vi "Line Detector.vi"(6 "milliseconds to wait":u32=100, 8 "error in":errorcluster, 9 "kena brp":dbl, 10 "Speed":dbl=250.0, 11 "FPGA VI Reference Out 2":refnum<k20>) -> (0 "error out":errorcluster, 2 "STOP?":bool, 3 "FPGA VI Reference Out":refnum<k20>)   [LabVIEW 2019]
uses:
  <vilib>/Platform/TimedLoop/XDataNode/timing_clust.ctl
  <vilib>/Platform/TimedLoop/XDataNode/nitl_modes.ctl
  <vilib>/Platform/TimedLoop/XDataNode/wakeup.ctl
  <vilib>/robotics/Steering/Mecanum Wheel/Roller Orientation.ctl
  <vilib>/robotics/Steering/Wheel/Wheel Parameters.ctl
  <vilib>/robotics/Steering/Wheel/Rotation Direction.ctl
  <vilib>/robotics/Steering/Mecanum Steering Frame/NI_Robotics_Mecanum Steering Frame.lvclass
  C:/Program Files (x86)/National Instruments/LabVIEW 2019/vi.lib/robotics/Steering/Steering Frame/NI_Robotics_Steering Frame.lvclass
  <vilib>/robotics/Steering/Mecanum Wheel/Create Mecanum Wheel.vi
  <vilib>/robotics/Steering/Mecanum Steering Frame/Create Mecanum Steering Frame.vi
  <vilib>/Utility/error.llb/Error Cluster From Error Code.vi
  <vilib>/rvi/errors/niLvFpgaAdjustHostInterfaceError.vi
  <vilib>/robotics/Steering/Steering Frame/Apply Steering Frame Velocity to Motors.vi
  <vilib>/platform/TimedLoop/XDataNode/XDataNode.xnode
  <vilib>/robotics/Steering/Create Steering Frame/NI_Robotics_Create Steering Frame.xnode
  <vilib>/robotics/Steering/Class Type Definitions/Mecanum Steering Frame.ctl
  <vilib>/rvi/interface/nirviReadWriteControl/nirviReadWriteControl.xnode
  <vilib>/robotics/Steering/Steering Frame/NI_Robotics_Steering Frame.lvclass
  NiFpgaLv.dll
  <vilib>/rvi/interface/Simulation/niFpgaSimulationCallBeginRW.vi
  <vilib>/Platform/TimedLoop/XDataNode/XDNodeRunTimeDep.lvlib
  <vilib>/robotics/Steering/Class Type Definitions/NI_Robotics_Steering Class Types.lvlib
  <vilib>/robotics/Steering/Wheel/NI_Robotics_Wheel.lvclass
  <vilib>/robotics/Steering/Mecanum Wheel/NI_Robotics_Mecanum Wheel.lvclass
  C:/Program Files (x86)/National Instruments/LabVIEW 2019/vi.lib/robotics/Steering/Special Steering Frame/NI_Robotics_Special Steering Frame.lvclass
  <vilib>/rvi/interface/nirviOpenFPGA/nirviOpenFPGA.xnode
  Collin's Project/FPGA Bitfiles/MRmecanum_FPGATarget_FPGAMainModified_TerasRobot_LKSN2021.lvbitx
  <vilib>/FPGAPlugInAG/myRIO-1900/niLvFpga_Open_myRIO-1900.vi
  <vilib>/rvi/interface/common/dynamic/niFpgaDynamicAddResources.vi
panel:
  out "Reset Button":bool
  out "LINE 2":bool
  out "LINE 1":bool
  out "now":dbl
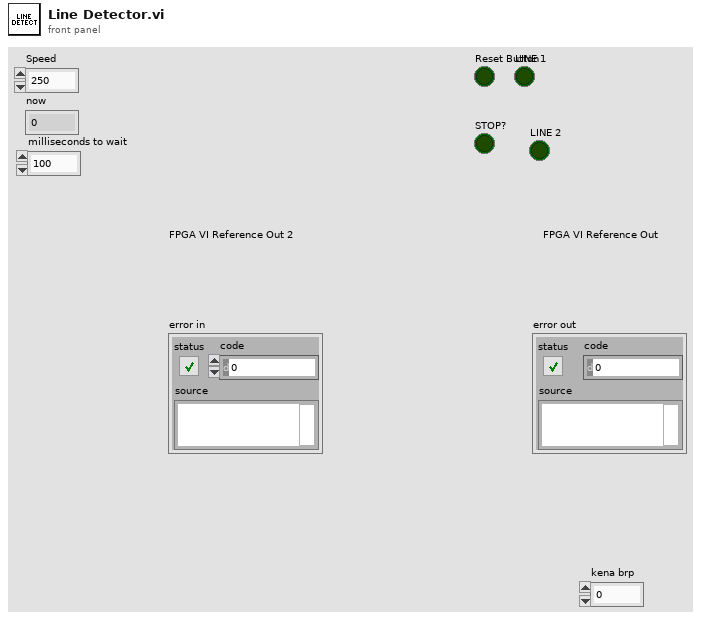
[diagram p1: front panel]
types:
  T1 = enum16{"maju", "mundur", "kanan", "kiri", "atas kanan", "atas kiri", "bawah kanan", "bawah kiri", "putar kanan", "putar kiri"}
  T2 = typedef "NI_Robotics_Steering Class Types.lvlib/Mecanum Steering Frame.ctl" = refnum<class "NI_Robotics_Mecanum Steering Frame.lvclass">
  T3 = typedef "XDNodeRunTimeDep.lvlib/timing_clust.ctl" = cluster{"Expected End [f-1]":u64, "Actual End [f-1]":u64, "Finished Late? [f-1]":bool, "Expected End [i-1]":u64, "Actual End [i-1]":u64, "Finished Late? [i-1]":bool, "Expected Start [i]":u64, "Actual Start [i]":u64, "Expected Start [f]":u64, "Actual Start [f]":u64, "Source Name":string, "Structure Name":string, "Period":i64, "Deadline":i64, "Offset":i64, "Start":i64, "Priority":i32, "Timeout":i32, "Mode":T4, "Wakeup Reason":T5, "Error":errorcluster, "Source Type":string, "Secondary Source Type":string, "Global End Time":u64, "Global Start Time":u64, "Frame Duration":u64, "Iteration Duration":u64, "Assigned CPU":i32, "I/O Scan Engine Mode":u32}
  T4 = typedef "XDNodeRunTimeDep.lvlib/nitl_modes.ctl" = enum32{"No Change", "Process missed periods, maintain original phase", "Discard missed periods, maintain original phase", "Process missed periods, ignore original phase", "Discard missed periods, ignore original phase"}
  T5 = typedef "XDNodeRunTimeDep.lvlib/wakeup.ctl" = enum32{"Normal", "Aborted", "Asynchronous wakeup", "Timing source error", "Timed loop error", "Timeout"}
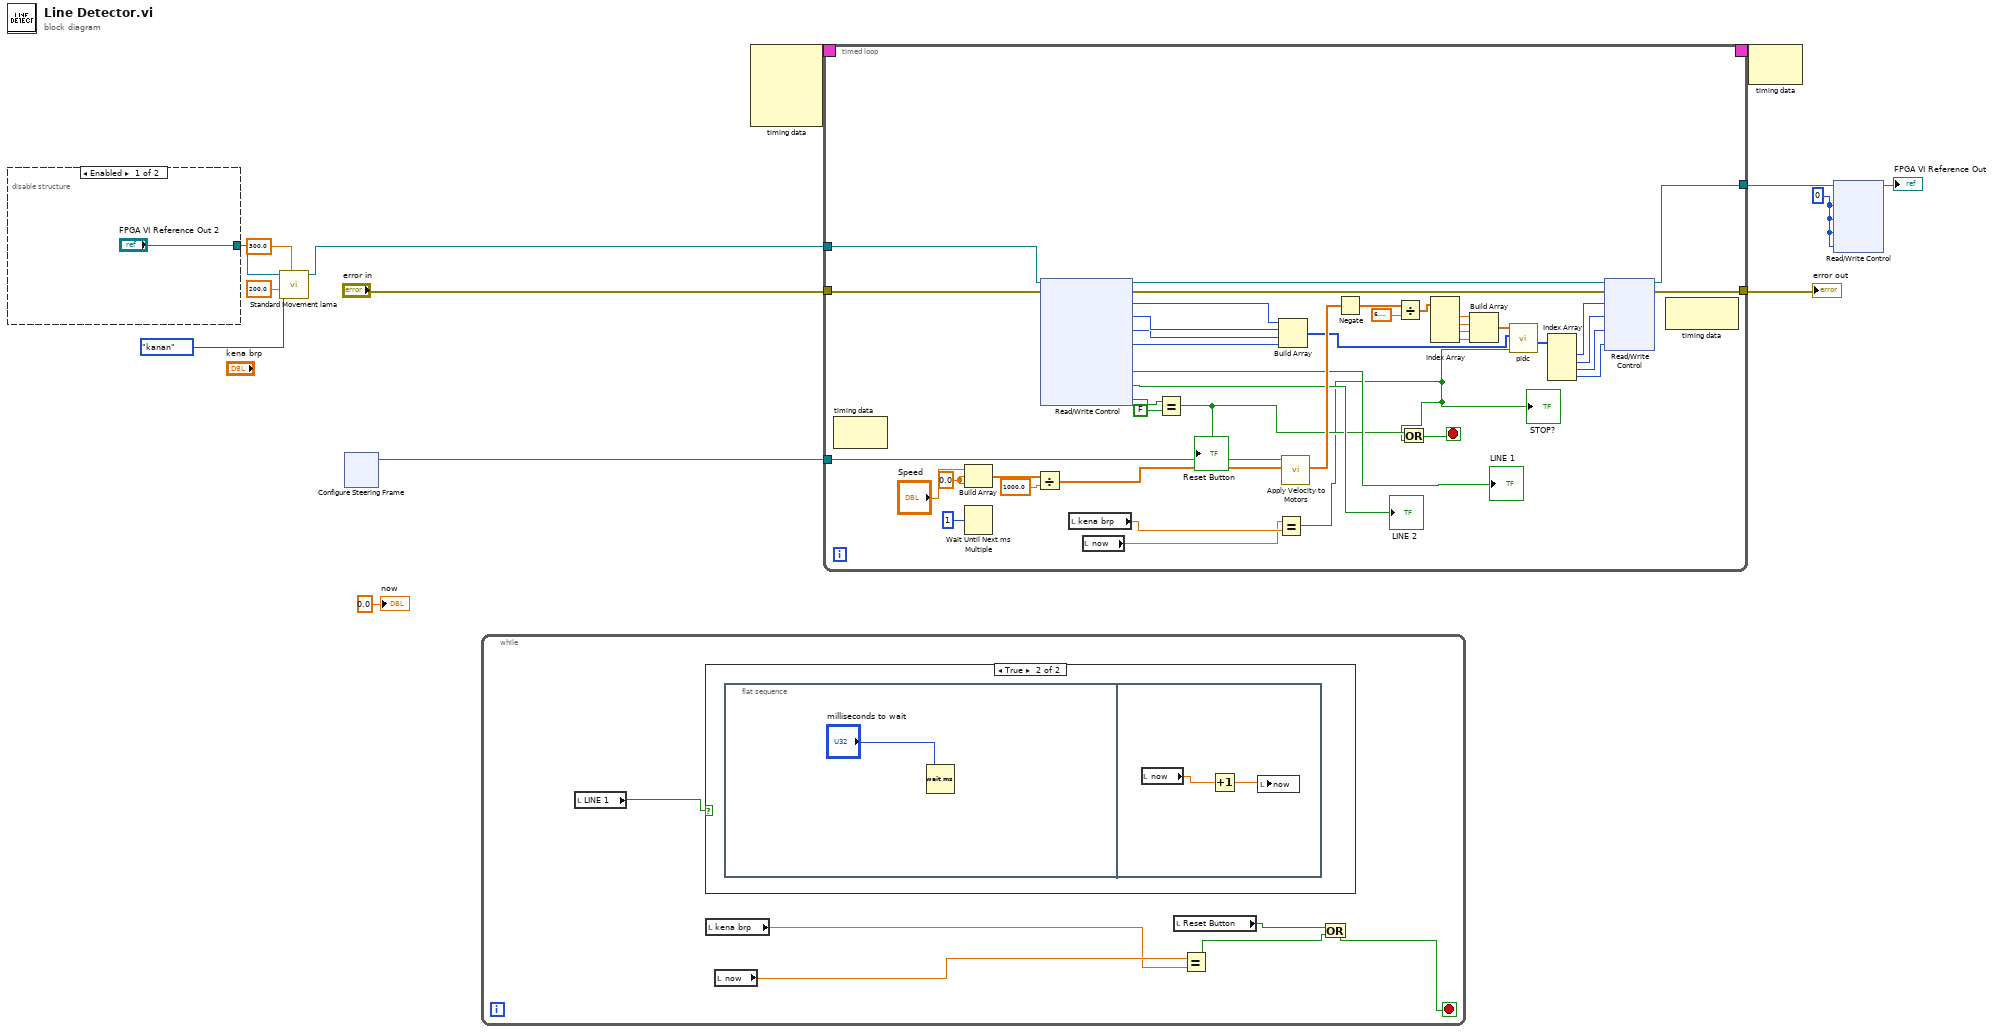
[diagram p0: block diagram]
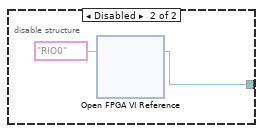
[diagram p3: hidden frame]
diagram:
  w7 = i16 0 ("M3")
  n1 = disable-structure shown="Enabled" {
    disable-tunnel: ["FPGA VI Reference Out 2" w16] -> w5
    frame Enabled {
    }
    frame Disabled {
      n2 = xnode "Open FPGA VI Reference"("resource name"=tag "RIO0") -> ("FPGA VI Reference Out"=w16:refnum<k20>)  [unwired: 1 in, 1 out]
    }
  }
  n3 = call "Standard Movement lama.vi"("Time"=300.0, "Speed"=200.0, "Move"=T1."kanan", "FPGA VI Reference Out 2"=w5) -> ("FPGA VI Reference Out"=w4:refnum<k20>)  [unwired: 6 in, 1 out]
  n4 = xnode ("Configure Steering Frame")() -> ("mecanum steering frame out"=w11:T2)  [unwired: 1 in, 1 out]
  n5 = while {
    stop <- w18 stop-if-true
    n6 = local read "LINE 1"() -> (w21:bool)
    n7 = case shown="True" w21 {
      frame False {
      }
      frame True {
        n8 = flat-sequence {
          frame #0 {
            n9 = Wait (ms)(milliseconds to wait="milliseconds to wait") -> ()  [unwired: 1 out]
          }
          frame #1 {
            n10 = local read "now"() -> (w26:dbl)
            n11 = Increment(x=w26) -> (x+1=w25:dbl)
            n12 = local write "now"(w25) -> ()
          }
        }
      }
    }
    n13 = local read "kena brp"() -> (w22:dbl)
    n14 = local read "now"() -> (w23:dbl)
    n15 = local read "Reset Button"() -> (w20:bool)
    n16 = Equal?(x=w23, y=w22) -> (x = y?=w19:bool)
    n17 = Or(x=w20, y=w19) -> (x .or. y?=w18:bool)
  }
  n18 = node-c288() -> (w13:T3)  [unwired: 4 in]
  n19 = timed-loop {
    timing: w13 -> [_]
    timing-out: [_] -> w12
    tunnel: w11 -> [w67]
    tunnel: w4 -> [w64]
    tunnel: [w66] -> w9
    tunnel: "error in" -> [w63]
    tunnel: [w65] -> w14
    stop <- w27 stop-if-true
    w37 = 0.0 ("element")
    n20 = node-c288() -> ()  [unwired: 1 in, 1 out]
    n21 = Build Array("Speed", w37, w37) -> (w41:dbl[])
    n22 = Wait Until Next ms Multiple(millisecond multiple=u32 1) -> ()  [unwired: 1 out]
    n23 = Divide(x=w41, y=1000.0) -> (x/y=w42:dbl[])
    n24 = xnode "Read/Write Control"("FPGA VI Reference In"=w64, "error in"=w63) -> ("FPGA VI Reference Out"=w36:refnum<k20>, "error out"=w61:errorcluster, "ENC M1"=w53:i32, "ENC M2"=w52:i32, "ENC M3"=w51:i32, "ENC M4"=w50:i32, "LINE 1"=→"LINE 1":bool, "LINE 2"=→"LINE 2":bool, "START BUTTON"=w31:bool)  [unwired: 1 out]
    n25 = local read "kena brp"() -> (w35:dbl)
    n26 = local read "now"() -> (w34:dbl)
    n27 = Equal?(x=w31, y=FALSE) -> (x = y?=w29:bool)
    "Reset Button" <- w29
    n28 = Equal?(x=w34, y=w35) -> (x = y?=w28:bool)
    "STOP?" <- w28
    n29 = Build Array(w53, w52, w51, w50) -> (w49:i32[])
    n30 = call-poly <vilib>:"Apply Velocity to Motors.vi"("steering frame velocity"=w42, "steering frame in"=w67) -> ("ccw motor velocity setpoints"=w62:dbl[])  [unwired: 5 in, 4 out]
    n31 = Negate(x=w62) -> (-x=w60:dbl[])
    n32 = Divide(x=w60, y=6.283185307179586) -> (x/y=w58:dbl[])
    n33 = Or(x=w29, y=w28) -> (x .or. y?=w27:bool)
    n34 = Index Array(array=w58) -> (element #1=w57:dbl, element #2=w56:dbl, element #3=w55:dbl, element #4=w54:dbl)  [unwired: 4 in]
    n35 = Build Array(w57, w56, w55, w54) -> (w48:dbl[])
    n36 = call "pidc.vi"("Stop"=w28, "input encoder 2"=w49, "input rps"=w48) -> ("Output duty cycle"=w47:i16[])  [unwired: 8 in]
    n37 = Index Array(array=w47) -> (element #1=w46:i16, element #2=w45:i16, element #3=w44:i16, element #4=w43:i16)  [unwired: 4 in]
    n38 = xnode "Read/Write Control"("FPGA VI Reference In"=w36, "error in"=w61, "M1"=w46, "M2"=w45, "M3"=w44, "M4"=w43) -> ("FPGA VI Reference Out"=w66:refnum<k20>, "error out"=w65:errorcluster)
    n39 = node-c288() -> ()  [unwired: 1 in, 1 out]
  }
  "error out" <- w14
  n40 = node-c288(w12) -> ()  [unwired: 1 out]
  n41 = xnode "Read/Write Control"("FPGA VI Reference In"=w9, "M3"=w7, "M1"=w7, "M4"=w7, "M2"=w7) -> ("FPGA VI Reference Out"=→"FPGA VI Reference Out":refnum<k20>)  [unwired: 1 in, 1 out]
  "now" <- 0.0 ("now")
